vi "sub vi - cycle&temp fail v6.vi"(0 "Amps Lo?":bool, 2 "Input Cluster":T1, 3 "SELECT":T2(ring), 4 "Amps Hi?":bool, 5 "Result In":bool) -> (15 "(FAIL) out":cluster{"FAIL LO":dbl, "FAIL HI":dbl}, 16 "(DISP) out":T3, 17 "T-RISE":cluster{"T-RISE (L)":dbl, "T-RISE (N)":dbl}, 18 "Result Out":bool, 19 "file error":errorcluster)   [LabVIEW 2013]
uses:
  program files/Global display 3.vi
  program files/Global 1.vi
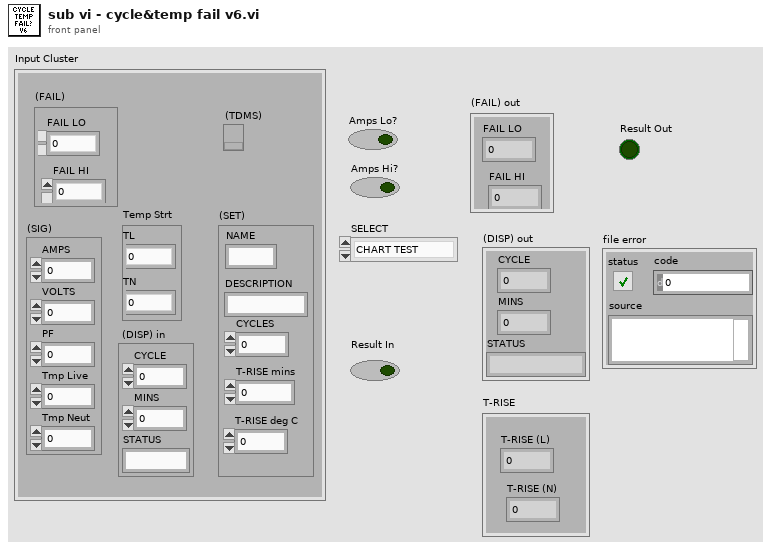
[diagram p1: front panel]
types:
  T1 = cluster{"(FAIL)":cluster{"FAIL LO":dbl, "FAIL HI":dbl}, "(SIG)":cluster{"AMPS":dbl, "VOLTS":dbl, "PF":dbl, "Tmp Live":dbl, "Tmp Neut":dbl}, "Temp Strt":cluster{"TL":dbl, "TN":dbl}, " (DISP) in":cluster{"CYCLE":dbl, "MINS":dbl, "STATUS":string}, "(SET)":cluster{"NAME":string, "DESCRIPTION":string, "CYCLES":dbl, "T-RISE mins":dbl, "T-RISE deg C":dbl}, "(TDMS)":refnum<k34>}
  T2 = enum32{"CHART TEST", "CYCLE TEST", "T-RISE TEST"}
  T3 = cluster{"CYCLE":dbl, "MINS":dbl, "STATUS":string}
  T4 = cluster{"AMPS":dbl, "VOLTS":dbl, "PF":dbl, "Tmp Live":dbl, "Tmp Neut":dbl}
  T5 = cluster{"NAME":string, "DESCRIPTION":string, "CYCLES":dbl, "T-RISE mins":dbl, "T-RISE deg C":dbl}
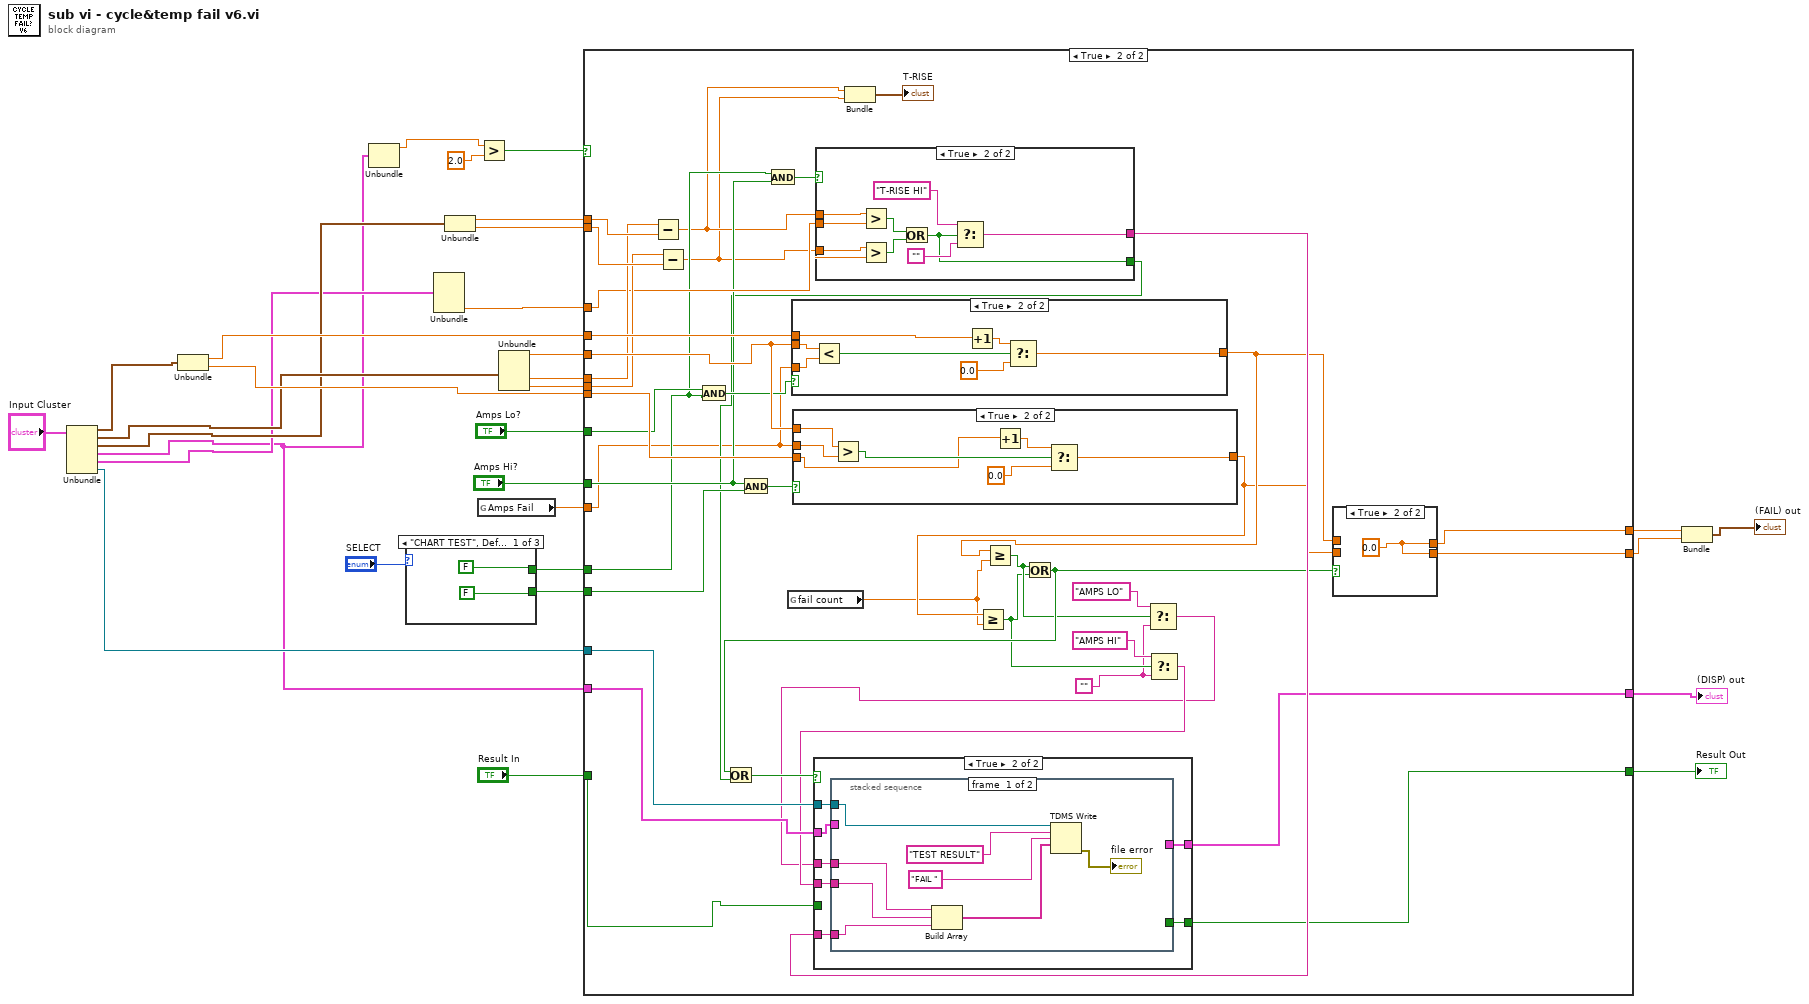
[diagram p0: block diagram]
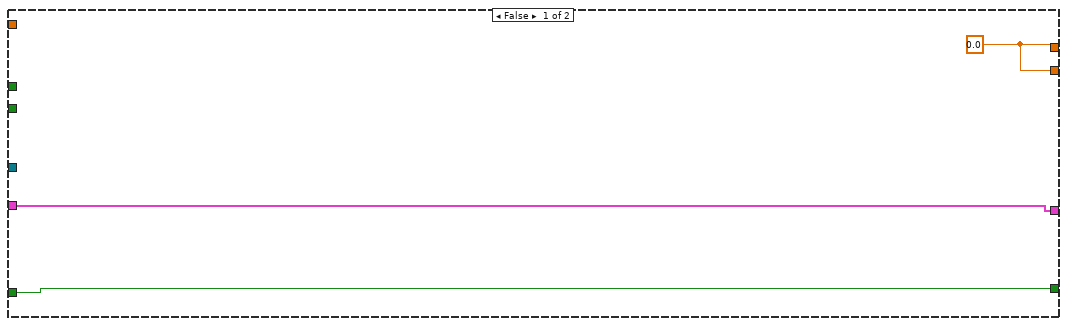
[diagram p2: hidden frame]
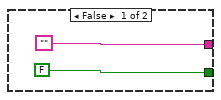
[diagram p4: hidden frame]
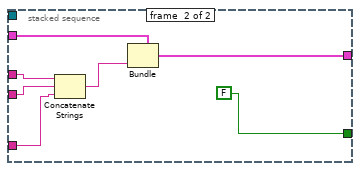
[diagram p6: hidden frame]
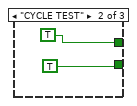
[diagram p9: hidden frame]
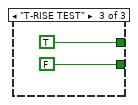
[diagram p10: hidden frame]
diagram:
  n1 = Unbundle("Input Cluster") -> ("(FAIL)"=w16:cluster{"FAIL LO":dbl, "FAIL HI":dbl}, "(SIG)"=w13:T4, "Temp Strt"=w12:cluster{"TL":dbl, "TN":dbl}, "(DISP) in"=w3:T3, "(SET)"=w11:T5, "(TDMS)"=w10:refnum<k34>)
  n2 = Unbundle(w16) -> ("FAIL LO"=w15:dbl, "FAIL HI"=w14:dbl)
  n3 = Unbundle(w3) -> ("CYCLE"=w2:dbl)  [unwired: 2 out]
  n4 = case shown="\"CHART TEST\", Default" "SELECT" {
    tunnel: [FALSE TRUE TRUE] -> w20
    tunnel: [FALSE TRUE FALSE] -> w23
    frame "CHART TEST", Default {
    }
    frame "CYCLE TEST" {
    }
    frame "T-RISE TEST" {
    }
  }
  n5 = Unbundle(w11) -> ("T-RISE deg C"=w24:dbl)  [unwired: 4 out]
  n6 = Unbundle(w12) -> ("TL"=w28:dbl, "TN"=w27:dbl)
  n7 = global read "Global display 3.vi" "Amps Fail"() -> (w1:dbl)
  n8 = Greater?(x=w2, y=2.0) -> (0:w18:bool)
  n9 = Unbundle(w13) -> ("AMPS"=w29:dbl, "Tmp Live"=w26:dbl, "Tmp Neut"=w25:dbl)  [unwired: 2 out]
  n10 = case shown="True" w18 {
    tunnel: w29 -> [_ w79]
    tunnel: w15 -> [_ w78]
    tunnel: w14 -> [_ w77]
    tunnel: w10 -> [_ w76]
    tunnel: w3 -> [w38 w75]
    tunnel: w28 -> [_ w74]
    tunnel: w27 -> [_ w73]
    tunnel: w26 -> [_ w72]
    tunnel: w25 -> [_ w71]
    tunnel: w24 -> [_ w70]
    tunnel: w23 -> [_ w67]
    tunnel: "Amps Lo?" -> [_ w65]
    tunnel: "Amps Hi?" -> [_ w63]
    tunnel: w20 -> [_ w62]
    tunnel: [w39 w59] -> w8
    tunnel: [w39 w58] -> w7
    tunnel: [w38 w57] -> w6
    tunnel: [w37 w56] -> w5
    tunnel: "Result In" -> [w37 w55]
    tunnel: w1 -> [_ w40]
    frame False {
      w39 = 0.0
    }
    frame True {
      w47 = ""
      n11 = Subtract(x=w72, y=w74) -> (x-y=w44:dbl)
      n12 = Subtract(x=w71, y=w73) -> (x-y=w43:dbl)
      n13 = And(x=w65, y=w62) -> (x .and. y?=w66:bool)
      n14 = And(x=w63, y=w67) -> (x .and. y?=w68:bool)
      n15 = And(x=w62, y=w63) -> (x .and. y?=w64:bool)
      n16 = global read "Global 1.vi" "fail count"() -> (w41:dbl)
      n17 = case shown="True" w66 {
        tunnel: w79 -> [_ w133]
        tunnel: w40 -> [_ w132]
        tunnel: w78 -> [w126 w128]
        tunnel: [w126 w127] -> w61
        frame False {
        }
        frame True {
          n18 = Less?(x=w133, y=w132) -> (x < y?=w131:bool)
          n19 = Increment(x=w128) -> (x+1=w130:dbl)
          n20 = Select(t=w130, s=w131, f=0.0) -> (s? t:f=w127:dbl)
        }
      }
      n21 = case shown="True" w68 {
        tunnel: w79 -> [_ w125]
        tunnel: w40 -> [_ w124]
        tunnel: [w118 w120] -> w60
        tunnel: w77 -> [w118 w119]
        frame False {
        }
        frame True {
          n22 = Greater?(x=w125, y=w124) -> (0:w123:bool)
          n23 = Increment(x=w119) -> (x+1=w122:dbl)
          n24 = Select(t=w122, s=w123, f=0.0) -> (s? t:f=w120:dbl)
        }
      }
      n25 = case shown="True" w64 {
        tunnel: w70 -> [_ w93]
        tunnel: w44 -> [_ w86]
        tunnel: w43 -> [_ w85]
        tunnel: ["" w88] -> w69
        tunnel: [FALSE w87] -> w53
        frame False {
        }
        frame True {
          n26 = Greater?(x=w86, y=w93) -> (0:w91:bool)
          n27 = Greater?(x=w85, y=w93) -> (0:w92:bool)
          n28 = Or(x=w91, y=w92) -> (x .or. y?=w87:bool)
          n29 = Select(t="T-RISE HI", s=w87, f="") -> (s? t:f=w88:string)
        }
      }
      n30 = Bundle(w44, w43) -> (→"T-RISE":cluster{dbl, dbl})  [unwired: 1 in]
      n31 = Greater Or Equal?(x=w60, y=w41) -> (x >= y?=w50:bool)
      n32 = Greater Or Equal?(x=w61, y=w41) -> (x >= y?=w51:bool)
      n33 = Or(x=w51, y=w50) -> (x .or. y?=w54:bool)
      n34 = Or(x=w54, y=w53) -> (x .or. y?=w52:bool)
      n35 = Select(t="AMPS LO", s=w51, f=w47) -> (s? t:f=w45:string)
      n36 = Select(t="AMPS HI", s=w50, f=w47) -> (s? t:f=w46:string)
      n37 = case shown="True" w52 {
        tunnel: w45 -> [_ w102]
        tunnel: w46 -> [_ w101]
        tunnel: w75 -> [w95 w100]
        tunnel: w76 -> [_ w99]
        tunnel: w69 -> [_ w98]
        tunnel: [w95 w97] -> w57
        tunnel: [w94 w96] -> w56
        tunnel: w55 -> [w94 _]
        frame False {
        }
        frame True {
          n38 = stacked-sequence {
            tunnel: w102 -> [w103 w117]
            tunnel: w101 -> [w104 w116]
            tunnel: w100 -> [_ w114]
            tunnel: w99 -> [w106 _]
            tunnel: w98 -> [w105 w113]
            tunnel: [_ w112] -> w97
            tunnel: [_ FALSE] -> w96
            frame #0 {
              n39 = Build Array(w103, w104, w105) -> (w109:string[])
              n40 = TDMS Write(0:w106, 5:"TEST RESULT", 7:"FAIL ", 9:w109) -> (15:→"file error":errorcluster)  [unwired: 2 in, 3 out]
            }
            frame #1 {
              n41 = Concatenate Strings(w117, w116, w113) -> (w115:string)
              n42 = Bundle(cluster=w114, "STATUS"=w115) -> (w112:T3)  [unwired: 2 in]
            }
          }
        }
      }
      n43 = case shown="True" w54 {
        tunnel: w61 -> [w81 _]
        tunnel: w60 -> [w80 _]
        tunnel: [w81 w82] -> w59
        tunnel: [w80 w82] -> w58
        frame False {
        }
        frame True {
          w82 = 0.0
        }
      }
    }
  }
  "(DISP) out" <- w6
  "Result Out" <- w5
  n44 = Bundle("FAIL LO"=w8, "FAIL HI"=w7) -> (→"(FAIL) out":cluster{"FAIL LO":dbl, "FAIL HI":dbl})  [unwired: 1 in]
